vi "GetAttrib.vi"(0 "QuickSilver in":refnum<class "QuickSilver.lvclass">, 11 "error in (no error)":errorcluster) -> (1 "Mec NegLim":string, 2 "Mec PosLim":string, 3 "Mec Speed":dbl, 4 "QuickSilver out":refnum<class "QuickSilver.lvclass">, 5 "Mec ID":string, 6 "MecTargets":dbl[](array[numeric])=[0.0, 4.0, 34.0, 64.5, 95.0, 125.5], 7 "MecOffset":string, 8 "MecTarget":dbl caption="Target" min=-1.0 max=131.0 step=0.001 format="%.2f", 10 "VISA Mec":refnum<visa-resource-name>="COM6", 12 "MecEnabled":bool=TRUE, 13 "Mec Factor":dbl, 14 "Mec Acceleration":dbl, 15 "error out":errorcluster)   [LabVIEW 2012, in "QuickSilver.lvclass"]
uses:
  QuickSilver.lvclass
  QuickSilver.lvclass/QuickSilver.ctl
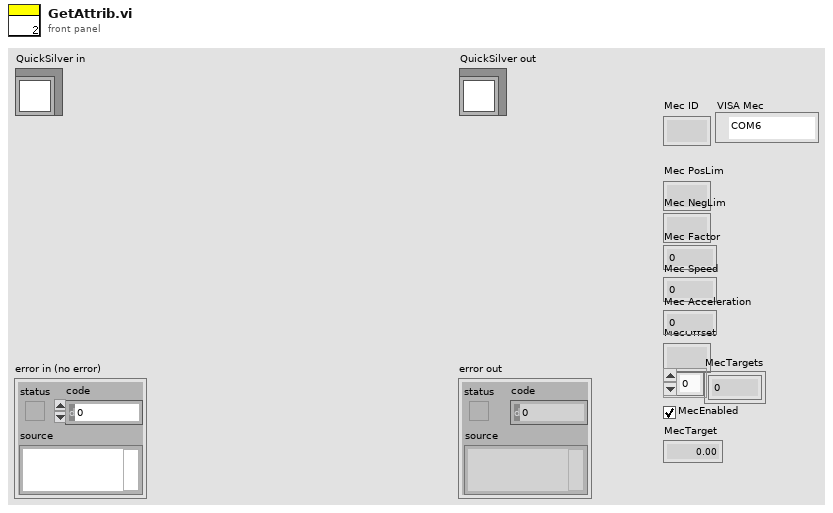
[diagram p1: front panel]
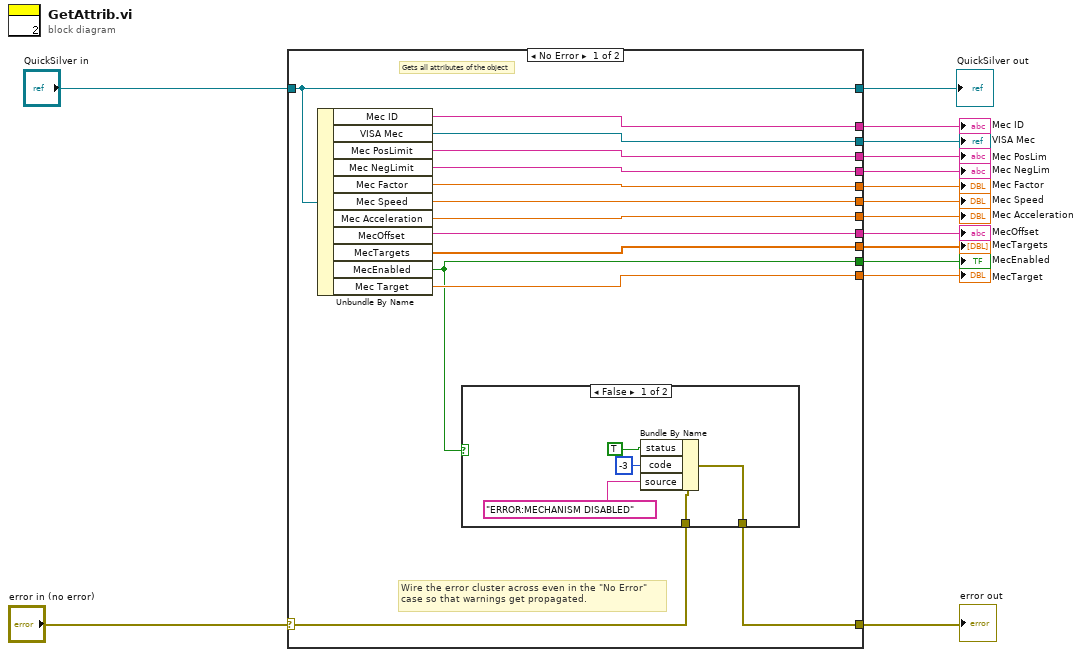
[diagram p0: block diagram]
diagram:
  n1 = case shown="No Error" "error in (no error)" {
    selector: "error in (no error)" -> [w18 w37]
    tunnel: [w17 w37] -> w1
    tunnel: [w29 w36] -> w3
    tunnel: "QuickSilver in" -> [w29 w36]
    tunnel: [w28 _] -> w15
    tunnel: [w27 _] -> w14
    tunnel: [w26 _] -> w13
    tunnel: [w25 _] -> w12
    tunnel: [w24 _] -> w11
    tunnel: [w23 _] -> w10
    tunnel: [w22 _] -> w9
    tunnel: [w21 _] -> w8
    tunnel: [w20 _] -> w7
    tunnel: [w16 _] -> w6
    tunnel: [w19 _] -> w5
    frame No Error {
      # "Gets all attributes of the object"
      # "Wire the error cluster across even in the \"No Error\"\ncase so that warnings get propagated."
      n2 = Unbundle By Name(w29) -> ("Mec ID"=w28:string, "VISA Mec"=w27:refnum<visa-resource-name>, "Mec PosLimit"=w26:string, "Mec NegLimit"=w25:string, "Mec Factor"=w24:dbl, "Mec Speed"=w23:dbl, "Mec Acceleration"=w22:dbl, "MecOffset"=w21:string, "MecTargets"=w20:dbl[], "MecEnabled"=w16:bool, "Mec Target"=w19:dbl)
      n3 = case shown="False" w16 {
        tunnel: w18 -> [w34 w35]
        tunnel: [w33 w35] -> w17
        frame False {
          n4 = Bundle By Name(cluster=w34, "status"=TRUE, "code"=-3, "source"="ERROR:MECHANISM DISABLED") -> (w33:errorcluster)
        }
        frame True {
        }
      }
    }
    frame Error {
      # "Error detected earlier: bypass"
    }
  }
  "error out" <- w1
  "QuickSilver out" <- w3
  "Mec ID" <- w15
  "Mec PosLim" <- w13
  "Mec NegLim" <- w12
  "MecOffset" <- w8
  "Mec Factor" <- w11
  "Mec Speed" <- w10
  "Mec Acceleration" <- w9
  "VISA Mec" <- w14
  "MecTargets" <- w7
  "MecEnabled" <- w6
  "MecTarget" <- w5
